vi "codetesting.vi"() -> ()   [LabVIEW 2015]
panel:
  in  "stop":bool
  out "Real 2":dbl
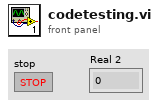
[diagram p1: front panel]
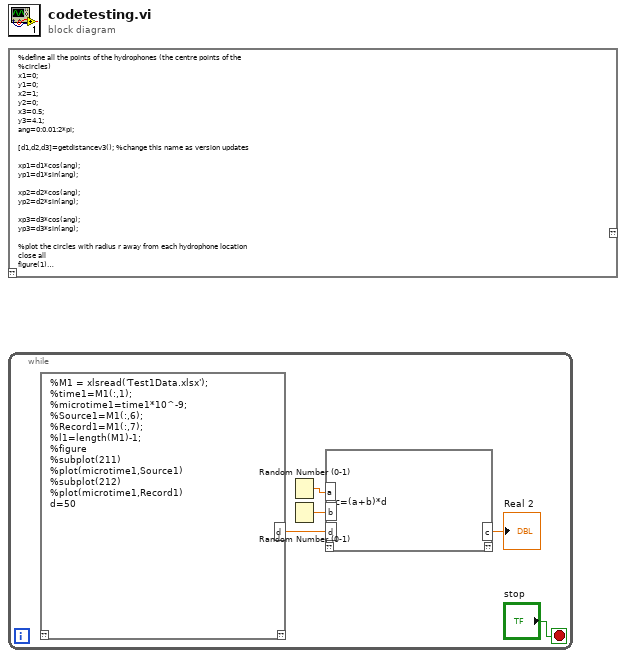
[diagram p0: block diagram]
diagram:
  n1 = script code="%define all the points of the hydrophones (the centre points of the\n%circles)\nx1=0;\ny1=0;\nx2=1;\ny2=0;\nx3=0.5;\ny3=4.1;\nang=0:0.01:2*pi;\n\n[d1,d2,d3]=getdistancev3(); %change this name as version updates\n\nxp1=d1*cos(ang);\nyp1=d1*sin(ang);\n\nxp2=d2*cos(ang);\nyp2=d2*sin(ang);\n\nxp3=d3*cos(ang);\nyp3=d3*sin(ang);\n\n%plot the circles with radius r away from each hydrophone location\nclose all\nfigure(1)\nscatter(x1,y1,'c','d','filled')\nhold on\nscatter(x2,y2,'c','d','filled')\nhold on\nscatter(x3,y3,'c','d','filled')\nhold on\nplot(x1+xp1,y1+yp1,x2+xp2,y2+yp2,x3+xp3,y3+yp3) \nxlabel('X coordinate');\nylabel('Y coordinate');\nhold on\n\n%Calculate the points of intersection of the circles\n[xout12,yout12] = circcirc(x1,y1,d1,x2,y2,d2);\n[xout13,yout13] = circcirc(x1,y1,d1,x3,y3,d3);\n[xout23,yout23] = circcirc(x2,y2,d2,x3,y3,d3);\n\n%If there are 2 points of intersection between 2 circles, then there will\n%be 2 x-values and 2 y-values for each. xypos separates combines the xout\n%yout values into an array of all intersection points\nxypos =[xout12(1) yout12(1)\n    xout12(2) yout12(2)\n    xout13(1) yout13(1)\n    xout13(2) yout13(2)\n    xout23(1) yout23(1)\n    xout23(2) yout23(2)];\n%Separates the x coordinates and y coordinates into 1d arrays and plots\n%the intersection points on the same graph\nx=xypos(:,1);\ny=xypos(:,2);\nscatter(x,y);\n\n%Run function to find mean x and y coordinates of location\n[mx,my]=our_function(xypos)\n\n%Plot calculated position\nhold on\nscatter(mx,my,'r','filled')\ngrid on"() -> ()  [unwired: 1 in, 1 out]
  n2 = while {
    stop <- "stop" stop-if-true
    n3 = script code="%M1 = xlsread('Test1Data.xlsx');\n%time1=M1(:,1);\n%microtime1=time1*10^-9;\n%Source1=M1(:,6);\n%Record1=M1(:,7);\n%l1=length(M1)-1;\n%figure\n%subplot(211)\n%plot(microtime1,Source1)\n%subplot(212)\n%plot(microtime1,Record1)\nd=50"() -> ("d"=w1:dbl)  [unwired: 1 in, 1 out]
    n4 = Random Number (0-1)() -> (number: 0 to 1=w3:dbl)
    n5 = Random Number (0-1)() -> (number: 0 to 1=w2:dbl)
    n6 = script code="c=(a+b)*d"("a"=w3, "b"=w2, "d"=w1) -> ("c"=→"Real 2":dbl)  [unwired: 1 in, 1 out]
  }
